vi "PID with Noise Plant.vi"() -> ()   [LabVIEW 2023]
doc: "This example demonstrates how to simulate a general PID controller with a plant with noise."
uses:
  <vilib>/Analysis/3filter.llb/Filter Passband Type.ctl
  <vilib>/addons/control/pid/pid.llb/PID Control Input Filter (DBL).vi
  <vilib>/addons/control/pid/pid.llb/PID (DBL).vi
  <vilib>/addons/control/pid/pid.llb/PID Output Rate Limiter (DBL).vi
  <vilib>/addons/control/pid/NI_PID_pid.lvlib
  <vilib>/ptbypt/NI_PtbyPt.lvlib
  <vilib>/Analysis/NI_AALBase.lvlib
panel:
  out "Sampling frequency (Hz)":dbl=4.0
  in  "cut-off frequency":dbl=6.0
  in  "order":i32=5
  in  "Filtering option":T1(ring)
  out "Manipulated variable (MV)":dbl(graph)=44.75756470842677
  in  "Output Limiter":bool
  in  "Output Rate (EGU/min)":dbl=10000.0 format="%#.2f"
  out "Unfiltered PV:":dbl=55.83860880961906 format="%.4f"
  in  "SP:":dbl(slide)=55.55555555555556 min=0.0 max=0.0 scale=0.0..100.0
  out "MV:":dbl(slide)=38.025391430574594 scale=-100.0..100.0
  out "PV:":dbl(slide)=55.83860880961906 scale=0.0..100.0
  in  "Noise Level":dbl(slide)=2.0 scale=0.1..10.0
  in  "PID gains":T2={"proportional gain (Kc)"=10.0, "integral time (Ti, min)"=0.01, "derivative time (Td, min)"=0.0} {"derivative time (Td, min)" format="%.3f"; "integral time (Ti, min)" format="%.3f"; "proportional gain (Kc)" format="%.3f"}
  in  "Controller Sampling Time":dbl=0.25 min=0.001 step=0.01 format="%#.3p"
  in  "Stop":bool
  out "System Monitor":T3(graph)={"PV:"=55.13720442402905, "SP:"=55.55555555555556, "Process Variable (%)"=55.83860880961906}
  # "Overview: This example demonstrates how to simulate a simple PID controller in a plant with noise.\nInstructions:\n1. Run the VI and wait until it reaches steady-state (PV doesn't change).\n2. Select a Filtering options and verify how this affects the Manipulated Variable (MV) and its Process Variable (PV).\n3. Click the Output Rate checkbox and verify how this affects the controller. In general, the output limit will reduce big 'jumps' on the output signal.\n4. Click Stop to stop the VI."
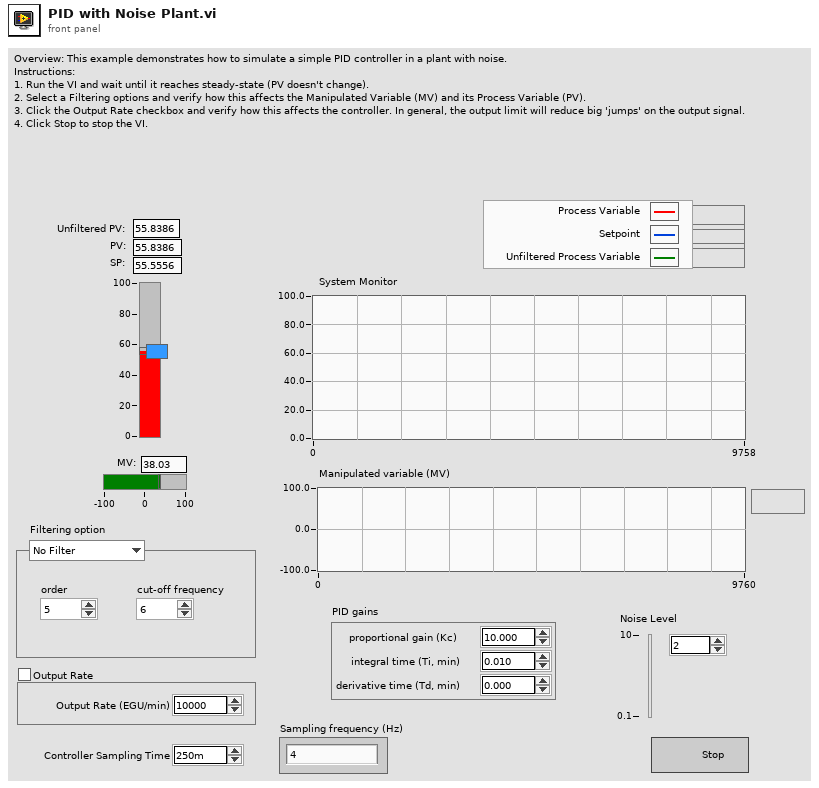
[diagram p1: front panel]
types:
  T1 = enum16{"No Filter", "PID FIR Filter", "Butterworth", "Chebyshev", "FIR Windowing", "Median"}
  T2 = cluster{"proportional gain (Kc)":dbl, "integral time (Ti, min)":dbl, "derivative time (Td, min)":dbl}
  T3 = cluster{"PV:":dbl, "SP:":dbl, "Process Variable (%)":dbl}
  T4 = typedef "NI_AALBase.lvlib/Filter Passband Type.ctl" = enum32{"Lowpass", "Highpass", "Bandpass", "Bandstop"}
  T5 = cluster{"static gain":dbl, "lag (min)":dbl, "dead cycles":dbl, "load %":dbl, "deadband":dbl, "noise level %":dbl, "initial PV":dbl, "initial PV 2":dbl}
  T6 = cluster{"PV:":dbl, "SP:":dbl, "Plant Output":dbl}
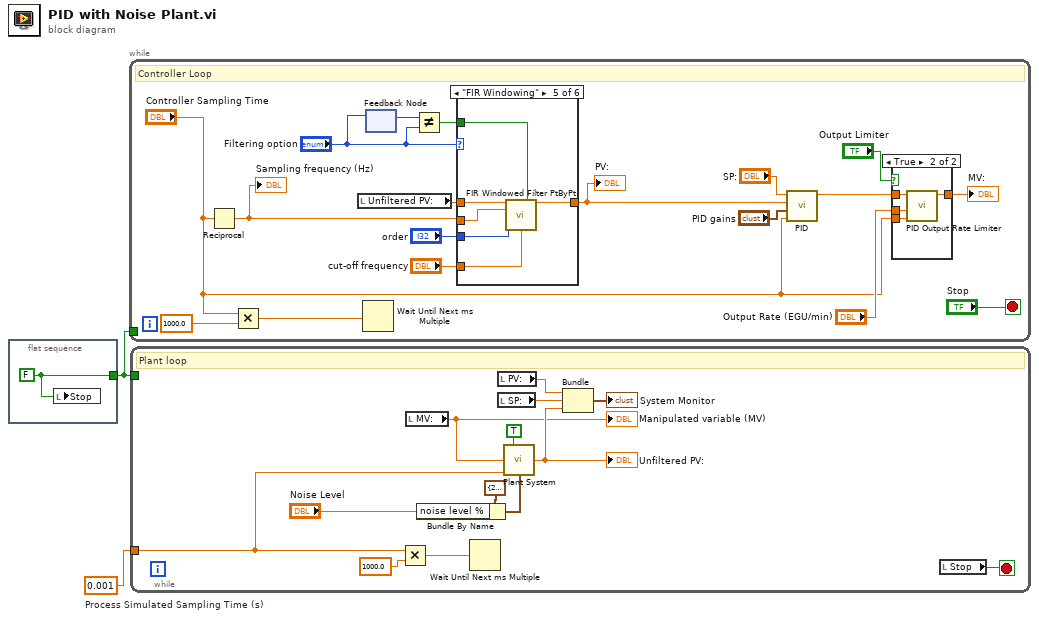
[diagram p0: block diagram]
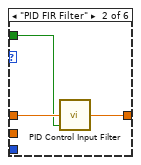
[diagram p3: hidden frame]
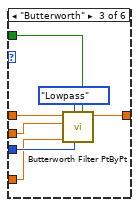
[diagram p4: hidden frame]
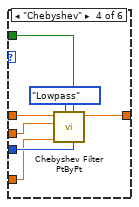
[diagram p5: hidden frame]
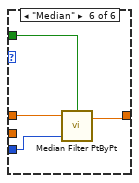
[diagram p6: hidden frame]
diagram:
  w2 = 0.001  # Process Simulated Sampling Time (s)
  n1 = flat-sequence {
    tunnel: [w3] -> w1
    frame #0 {
      w3 = FALSE ("STOP")
      n2 = local write "Stop"(w3) -> ()
    }
  }
  n3 = while {
    tunnel: w1 -> [_]
    stop <- "Stop" stop-if-true
    # "Controller Loop"
    n4 = Reciprocal(x="Controller Sampling Time") -> (1/x=w20:dbl)
    "Sampling frequency (Hz)" <- w20
    n5 = Multiply(x="Controller Sampling Time", y=1000.0) -> (x*y=w21:dbl)
    n6 = local read "Unfiltered PV:"() -> (w16:dbl)
    n7 = Wait Until Next ms Multiple(millisecond multiple=w21) -> ()  [unwired: 1 out]
    n8 = feedback-in #1("Filtering option") -> ()
    n9 = feedback #1() -> (w8:T1)  [unwired: 1 in]
    n10 = Not Equal?(x=w8, y="Filtering option") -> (x != y?=w6:bool)
    n11 = case shown="\"FIR Windowing\"" "Filtering option" {
      tunnel: [w22 w25 w32 w39 w45 w49] -> w17
      tunnel: w16 -> [w22 w24 w31 w38 w44 w48]
      tunnel: w20 -> [_ _ w30 w37 w43 _]
      tunnel: "order" -> [_ _ w28 w35 w42 w47]
      tunnel: "cut-off frequency" -> [_ _ w27 w34 w41 _]
      tunnel: w6 -> [_ w23 w26 w33 w40 w46]
      frame "No Filter", Default {
      }
      frame "PID FIR Filter" {
        n12 = call-poly <vilib>:"PID Control Input Filter.vi"("reinitialize? (F)"=w23, "input"=w24) -> ("output"=w25:dbl)  [unwired: 3 in]
      }
      frame "Butterworth" {
        n13 = call <vilib>:"Butterworth Filter PtByPt.vi"("initialize"=w26, "order"=w28, "filter type"=Filter_Passband_Type."Lowpass", "low cutoff freq: fl"=w27, "sampling freq: fs"=w30, "x"=w31) -> ("Filtered x"=w32:dbl)  [unwired: 3 in, 1 out]
      }
      frame "Chebyshev" {
        n14 = call <vilib>:"Chebyshev Filter PtByPt.vi"("order"=w35, "initialize"=w33, "filter type"=Filter_Passband_Type."Lowpass", "low cutoff freq: fl"=w34, "sampling freq: fs"=w37, "x"=w38) -> ("Filtered x"=w39:dbl)  [unwired: 4 in, 1 out]
      }
      frame "FIR Windowing" {
        n15 = call <vilib>:"FIR Windowed Filter PtByPt.vi"("x"=w44, "initialize"=w40, "sampling freq: fs"=w43, "taps"=w42, "low cutoff freq: fl"=w41) -> ("Filtered x"=w45:dbl)  [unwired: 9 in, 1 out]
      }
      frame "Median" {
        n16 = call <vilib>:"Median Filter PtByPt.vi"("initialize"=w46, "rank"=w47, "x"=w48) -> ("Filtered x"=w49:dbl)  [unwired: 1 in, 1 out]
      }
    }
    "PV:" <- w17
    n17 = call-poly <vilib>:"PID.vi"("dt (s)"="Controller Sampling Time", "PID gains"="PID gains", "process variable"=w17, "setpoint"="SP:") -> ("output"=w15:dbl)  [unwired: 6 in, 1 out]
    n18 = case shown="True" "Output Limiter" {
      tunnel: w15 -> [w50 w54]
      tunnel: "Controller Sampling Time" -> [_ w53]
      tunnel: [w50 w52] -> w14
      tunnel: "Output Rate (EGU/min)" -> [_ w51]
      frame False {
      }
      frame True {
        n19 = call-poly <vilib>:"PID Output Rate Limiter.vi"("dt (s)"=w53, "output rate (EGU/min)"=w51, "input (controller output)"=w54) -> ("output"=w52:dbl)  [unwired: 5 in, 1 out]
      }
    }
    "MV:" <- w14
  }
  n20 = while {
    tunnel: w2 -> [w59]
    tunnel: w1 -> [_]
    stop <- w63 stop-if-true
    # "Plant loop"
    n21 = Multiply(x=w59, y=1000.0) -> (x*y=w60:dbl)
    n22 = local read "MV:"() -> (w61:dbl)
    "Manipulated variable (MV)" <- w61
    n23 = Bundle By Name(cluster=T5 {"static gain"=2.5, "lag (min)"=18.0, "dead cycles"=0.0, "load %"=50.0, "deadband"=0.0, "noise level %"=0.1, "initial PV"=0.0, "initial PV 2"=0.0} ("process parameters 2"), "noise level %"="Noise Level") -> (w56:T5)
    n24 = Wait Until Next ms Multiple(millisecond multiple=w60) -> ()  [unwired: 1 out]
    n25 = local read "PV:"() -> (w64:dbl)
    n26 = local read "SP:"() -> (w66:dbl)
    n27 = call "Plant System.vi"("Integrator ?"=TRUE, "Plant Input"=w61, "dt (s)"=w59, "process parameters"=w56) -> ("Plant Output"=w62:dbl)  [unwired: 11 in]
    "Unfiltered PV:" <- w62
    n28 = Bundle("PV:"=w64, "SP:"=w66, "Plant Output"=w62) -> (→"System Monitor":T6)  [unwired: 1 in]
    n29 = local read "Stop"() -> (w63:bool)
  }
